vi "FA_Create_New_Events.vi"(8 "error in":errorcluster, 11 "XML String":string) -> (0 "error out":errorcluster)   [LabVIEW 2013, in "FA_FIRST.lvlib"]
uses:
  FA_FIRST.lvlib
  Backend/source/VI Source/FRCts20_Backend_API/FRCts20_Backend_API_EventRoot.ctl
  FIRST Client/source/VI Source/FC_Competition Attributes.ctl
  Backend/source/VI Source/FRCts20_Backend_API/FRCts20_Backend_API_Command_EventRoot.ctl
  Backend/source/VI Source/FRCts20_Backend_API/FRCts20_Backend_API_EventRoot.vi
  FIRST Client/source/VI Source/FC_FIRST Client.lvlib
  Backend/source/VI Source/FRCts20_Backend_API/FRCts20_Backend_API.lvlib
panel:
  out "EventRoot In":T1
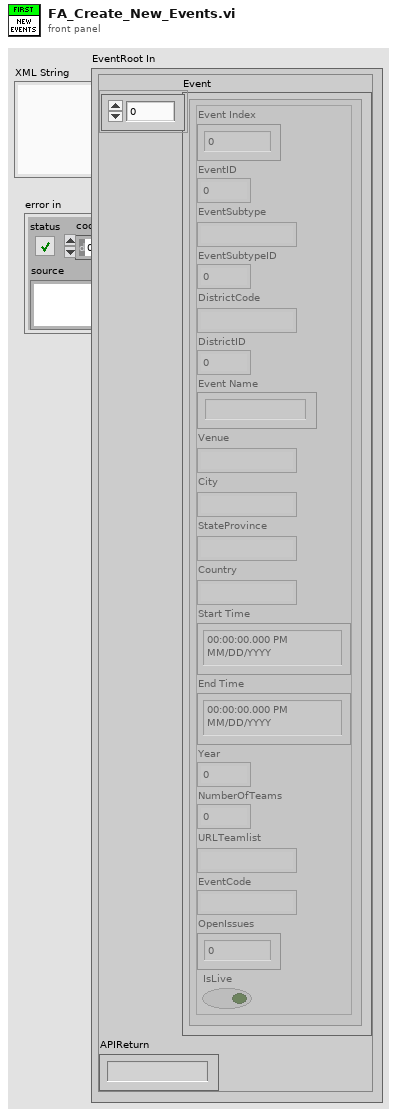
[diagram p1: front panel]
types:
  T1 = typedef "FRCts20_Backend_API.lvlib/FRCts20_Backend_API_EventRoot.ctl" = cluster{"Event":cluster{"Event Index":u32, "EventID":u32, "EventSubtype":string, "EventSubtypeID":u32, "DistrictCode":string, "DistrictID":u32, "Event Name":string, "Venue":string, "City":string, "StateProvince":string, "Country":string, "Start Time":timestamp, "End Time":timestamp, "Year":u32, "NumberOfTeams":u32, "URLTeamlist":string, "EventCode":string, "OpenIssues":u8, "IsLive":bool}[], "APIReturn":string}
  T2 = typedef "FRCts20_Backend_API.lvlib/FRCts20_Backend_API_Command_EventRoot.ctl" = string
  T3 = typedef "FC_FIRST Client.lvlib/FC_Competition Attributes.ctl" = cluster{"Event ID":string, "Event Subtype":string, "ID Event Subtype":string, "District Code":string, "ID District":string, "Event Name":string, "Venue":string, "City":string, "State":string, "Country":string, "Start Date":string, "End Date":string, "Year":string, "Number of Teams":string, "URL of Teamlist":string, "Event Code":string}
  T4 = cluster{"Event Index":u32, "EventID":u32, "EventSubtype":string, "EventSubtypeID":u32, "DistrictCode":string, "DistrictID":u32, "Event Name":string, "Venue":string, "City":string, "StateProvince":string, "Country":string, "Start Time":timestamp, "End Time":timestamp, "Year":u32, "NumberOfTeams":u32, "URLTeamlist":string, "EventCode":string, "OpenIssues":u8, "IsLive":bool}[]
  T5 = cluster{"Event Index":u32, "EventID":u32, "EventSubtype":string, "EventSubtypeID":u32, "DistrictCode":string, "DistrictID":u32, "Event Name":string, "Venue":string, "City":string, "StateProvince":string, "Country":string, "Start Time":timestamp, "End Time":timestamp, "Year":u32, "NumberOfTeams":u32, "URLTeamlist":string, "EventCode":string, "OpenIssues":u8, "IsLive":bool}
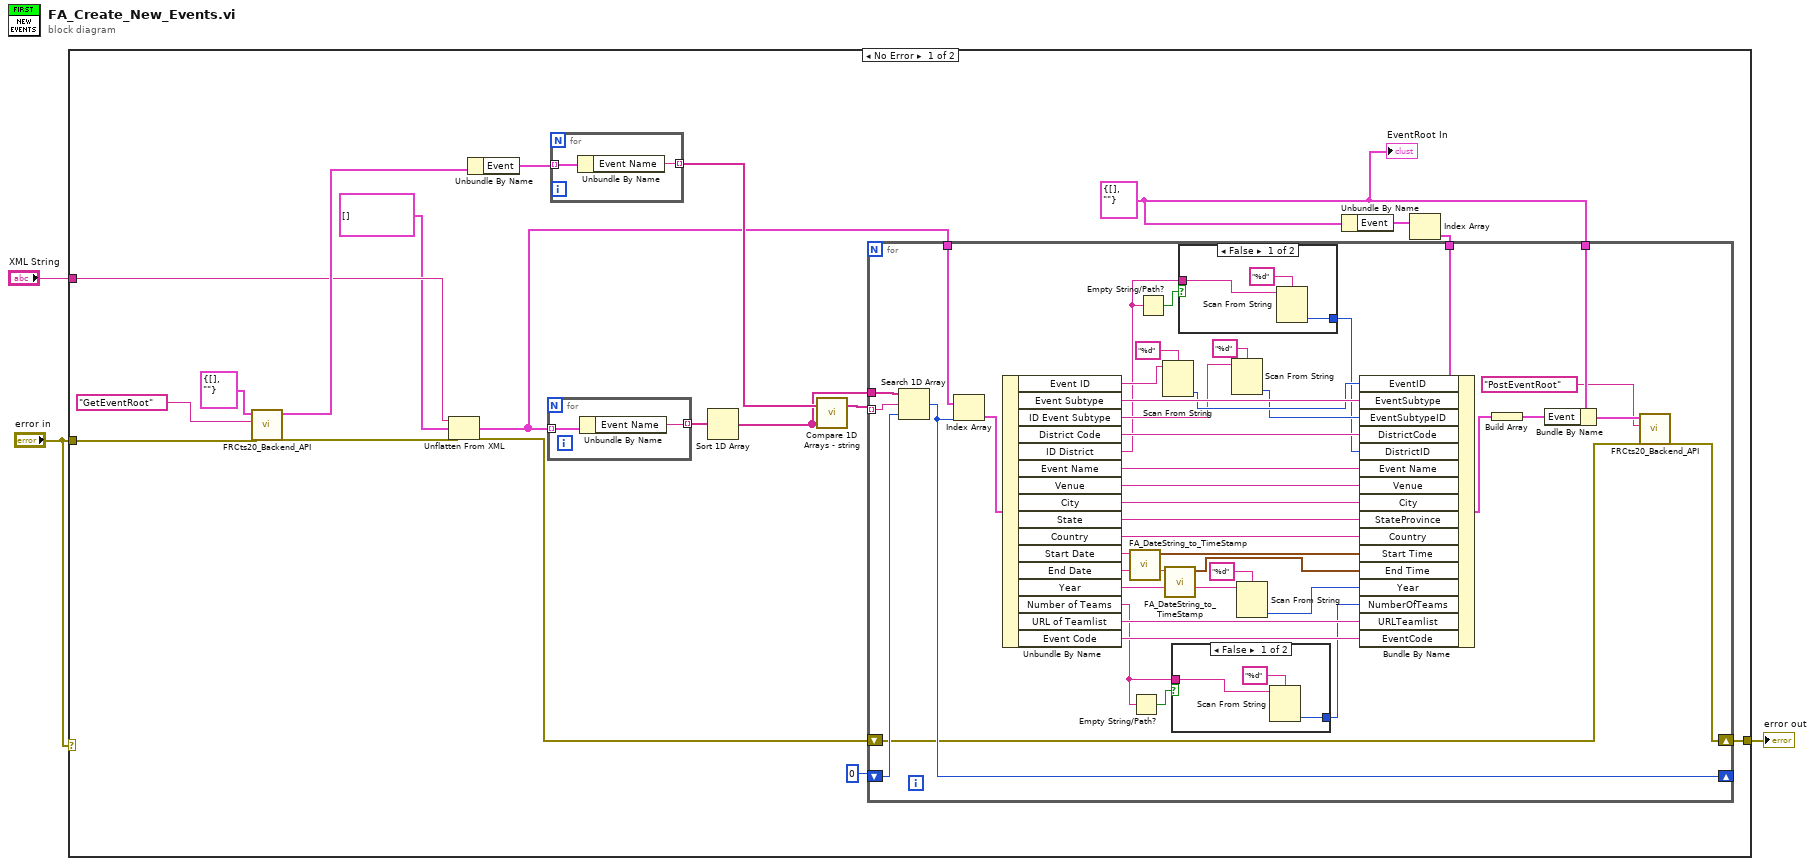
[diagram p0: block diagram]
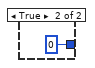
[diagram p2: hidden frame]
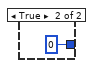
[diagram p3: hidden frame]
diagram:
  n1 = case shown="No Error" "error in" {
    tunnel: [w22 _] -> w3
    tunnel: "XML String" -> [w15 _]
    tunnel: "error in" -> [w10 _]
    frame No Error {
      w6 = T1 {"Event"=[], "APIReturn"=""} ("EventRoot In")
      n2 = call-poly "FRCts20_Backend_API.vi"("error in (no error)"=w10, "Message"=T2 "GetEventRoot", "EventRoot In"=T1 {"Event"=[], "APIReturn"=""}) -> ("error out"=w17:errorcluster, "EventRoot Out"=w21:T1)  [unwired: 6 in, 1 out]
      n3 = Unflatten From XML(xml string=w15, type=T3[] [], error in (no error)=w17) -> (value=w7:T3[], error out=w16:errorcluster)
      n4 = Unbundle By Name(w21) -> ("Event"=w5:T4)
      n5 = for {
        tunnel: w7 -> [w74] mode=indexing
        tunnel: [w73] -> w12 mode=indexing
        n6 = Unbundle By Name(w74) -> ("Event Name"=w73:string)
      }
      n7 = for {
        tunnel: [w76] -> w19 mode=indexing
        tunnel: w5 -> [w75] mode=indexing
        n8 = Unbundle By Name(w75) -> ("Event Name"=w76:string)
      }
      n9 = Sort 1D Array(array=w12) -> (sorted array=w8:string[])
      n10 = call "Compare 1D Arrays - string.vi"("New Array"=w8, "Old Array"=w19) -> ("Added"=w11:string[])  [unwired: 1 out]
      n11 = Unbundle By Name(w6) -> ("Event"=w4:T4)
      n12 = Index Array(array=w4) -> (element=w20:T5)  [unwired: 1 in]
      n13 = for {
        shift-right: [w63] -> _
        shift-left: 0 ("index of element") -> [w64]
        tunnel: w11 -> [w60] mode=indexing
        tunnel: w7 -> [w62]
        shift-right: [w57] -> w22
        shift-left: w16 -> [w56]
        tunnel: w20 -> [w58]
        tunnel: w6 -> [w55]
        tunnel: w8 -> [w51]
        n14 = Search 1D Array(1D array=w51, element=w60, start index (0)=w64) -> (index of element=w63:i32)
        n15 = Index Array(array=w62, index=w63) -> (element=w61:T3)
        n16 = Unbundle By Name(w61) -> ("Event ID"=w37:string, "Event Subtype"=w47:string, "ID Event Subtype"=w34:string, "District Code"=w46:string, "ID District"=w27:string, "Event Name"=w48:string, "Venue"=w50:string, "City"=w49:string, "State"=w42:string, "Country"=w43:string, "Start Date"=w41:string, "End Date"=w40:string, "Year"=w30:string, "Number of Teams"=w24:string, "URL of Teamlist"=w44:string, "Event Code"=w45:string)
        n17 = call "FA_DateString_to_TimeStamp.vi"("DateTime String"=w41) -> ("Time Stamp"=w39:timestamp)  [unwired: 10 in]
        n18 = Empty String/Path?(string/path=w24) -> (empty?=w25:bool)
        n19 = Empty String/Path?(string/path=w27) -> (empty?=w28:bool)
        n20 = Scan From String(format string="%d", input string=w37) -> (output 1=w36:i32)  [unwired: 3 in, 3 out]
        n21 = call "FA_DateString_to_TimeStamp.vi"("DateTime String"=w40) -> ("Time Stamp"=w26:timestamp)  [unwired: 10 in]
        n22 = case shown="False" w25 {
          tunnel: [w66 0] -> w23
          tunnel: w24 -> [w65 _]
          frame False {
            n23 = Scan From String(format string="%d", input string=w65) -> (output 1=w66:i32)  [unwired: 3 in, 3 out]
          }
          frame True {
          }
        }
        n24 = case shown="False" w28 {
          tunnel: [w70 0] -> w32
          tunnel: w27 -> [w69 _]
          frame False {
            n25 = Scan From String(format string="%d", input string=w69) -> (output 1=w70:i32)  [unwired: 3 in, 3 out]
          }
          frame True {
          }
        }
        n26 = Scan From String(format string="%d", input string=w34) -> (output 1=w33:i32)  [unwired: 3 in, 3 out]
        n27 = Scan From String(format string="%d", input string=w30) -> (output 1=w29:i32)  [unwired: 3 in, 3 out]
        n28 = Bundle By Name(cluster=w58, "EventID"=w36, "EventSubtype"=w47, "EventSubtypeID"=w33, "DistrictCode"=w46, "DistrictID"=w32, "Event Name"=w48, "Venue"=w50, "City"=w49, "StateProvince"=w42, "Country"=w43, "Start Time"=w39, "End Time"=w26, "Year"=w29, "NumberOfTeams"=w23, "URLTeamlist"=w44, "EventCode"=w45) -> (w59:T5)
        n29 = Build Array(w59) -> (w54:T4)
        n30 = Bundle By Name(cluster=w55, "Event"=w54) -> (w53:T1)
        n31 = call-poly "FRCts20_Backend_API.vi"("error in (no error)"=w56, "Message"=T2 "PostEventRoot", "EventRoot In"=w53) -> ("error out"=w57:errorcluster)  [unwired: 6 in, 2 out]
      }
      "EventRoot In" <- w6
    }
    frame Error {
    }
  }
  "error out" <- w3
